vi "ParametrosTeste.View.vi"() -> ()   [LabVIEW 2019]
uses:
  Telas.ctl
  <vilib>/Utility/miscctls.llb/LVStringsAndValuesArrayTypeDef_U16.ctl
  <vilib>/Utility/miscctls.llb/LVPositionTypeDef.ctl
  <vilib>/Utility/miscctls.llb/LVPointTypeDef.ctl
  TelaParametrosTeste/VariaveisParametros.vi
  TelaConfig/Configuracao.Variaveis.vi
  <vilib>/Utility/file.llb/Read Delimited Spreadsheet (DBL).vi
panel:
  out "OndaSelecionada":T1(ring)
  out "TipoGeraçãoSelect":u16(ring) items=["Modo Continuo", "Limitado por tempo", "Ponto por ponto"]
  out "HardwareConfiguration":T3(array[cluster])
  out "ProximaTela":T4
  in  "Tab":enum32{"Page 1", "Page 2"}(tab)
  in  "TabTela":enum32{"PlacaNI", "Geracao1", "Geracao2"}(tab)
  out "Info 2":string
  in  "EntradasAnalogicas":u16(ring) caption="Entrada Analógica:" items=["None"]
  in  "Placas":u16(ring) caption="Placa de aquisição:" items=["None"]
  in  "AddMedicao":bool caption="Adicionar:"
  in  "ListaMedicaoPorta":string[][](table)
  in  "TiposMedicoes":T5(ring) caption="Tipos de Medição:"
  out "GeracaoSelecionada":string
  in  "SelecionarGeracao":bool
  out "UnidadeTempoTeste":string
  in  "TempoTeste":dbl caption="Tempo do teste:"
  in  "TesteOnda":bool
  out "Graph":cluster{"X":dbl, "Y":dbl}[](graph)
  in  "TabOndas":T6(tab)
  in  "InfoContinuo":T7 {"TempRampas" format="%#_g s"}
  in  "InfoInSenoide":T8
  in  "Limpar pontos":bool
  in  "Pasta cvs":path caption="Pasta arquivo cvs:"
  in  "TaxaGeracao":dbl caption="Tempo entre pontos:"
  out "Pontos":dbl[](array[numeric]) caption="Pontos:"
  in  "SelectTipoOnda":T1(ring) caption="Forma de onda:"
  in  "Voltar":bool
  out "Info":string
  in  "BotaoProximaTela":bool
  in  "VoltarTela":bool
  in  "SelecaoGeracao":u16(ring) caption="Seleção forma de geração" items=["Modo Continuo", "Limitado por tempo", "Ponto por ponto"]
  in  "Salvar":bool
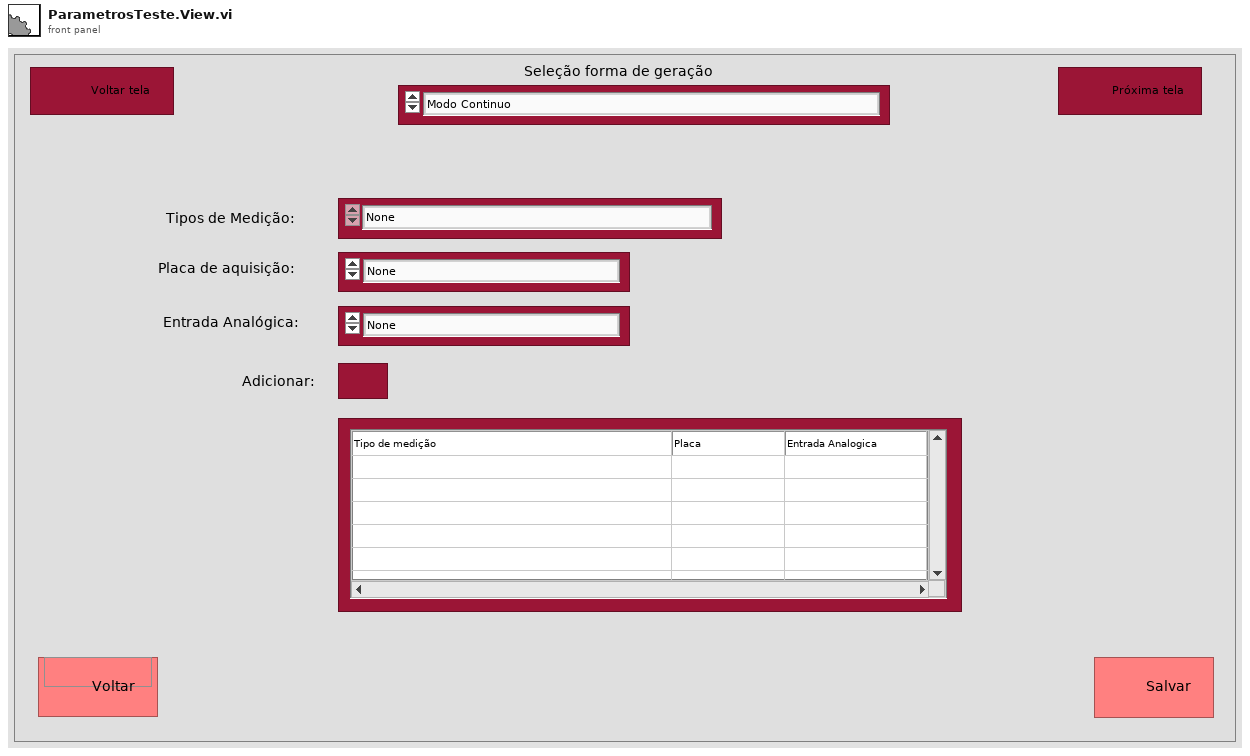
[diagram p1: front panel]
types:
  T1 = enum16{"None", "Continua", "Senoidal", "Quadrada"}
  T2 = typedef "LVStringsAndValuesArrayTypeDef_U16.ctl" = cluster{"String":string, "Value":u16}[]
  T3 = cluster{"ProductCategory":i32, "ProductType":string, "DevIsSimulated":bool, "DigitalInputs":tag[], "DigitalOutputs":tag[], "AnalogInputs":tag[], "AnalogOutputs":tag[], "AnalogInRing":T2}[]
  T4 = typedef "Telas.ctl" = enum16{"Selecao", "Config", "Medicao", "ParametrosTeste"}
  T5 = enum16{"None", "Tensão AeroGerador", "Corrente AeroGerador", "Anemômetro 1", "Anemômetro 2", "Vibração"}
  T6 = enum32{"Contino", "Senoide", "Pontos", "Quadrada"}
  T7 = cluster{"TempRampas":dbl, "PicoMax":dbl, "TextUnidMed":string}
  T8 = cluster{"TexPontosSenoide":string, "RotacaoMinuto":dbl, "PicoMin":dbl, "PicoMax":dbl, "TaxaGeracao":dbl}
  T9 = typedef "LVPositionTypeDef.ctl" = cluster{"Left":i32, "Top":i32}
  T10 = typedef "LVPointTypeDef.ctl" = cluster{"Horizontal":i16, "Vertical":i16}
  T11 = enum16{"None", "Continua", "Senoidal", "Quadrada", "Pontos"}
  T12 = cluster{"ProductCategory":i32, "ProductType":string, "DevIsSimulated":bool, "DigitalInputs":tag[], "DigitalOutputs":tag[], "AnalogInputs":tag[], "AnalogOutputs":tag[], "AnalogInRing":T2}
  T13 = cluster{"Texpontos senoide":string, "AceleracaoMaxima":dbl, "RotacaoMaxMotor":dbl, "PotenciaMotor":dbl, "AceleracaoMaxima 2":dbl}
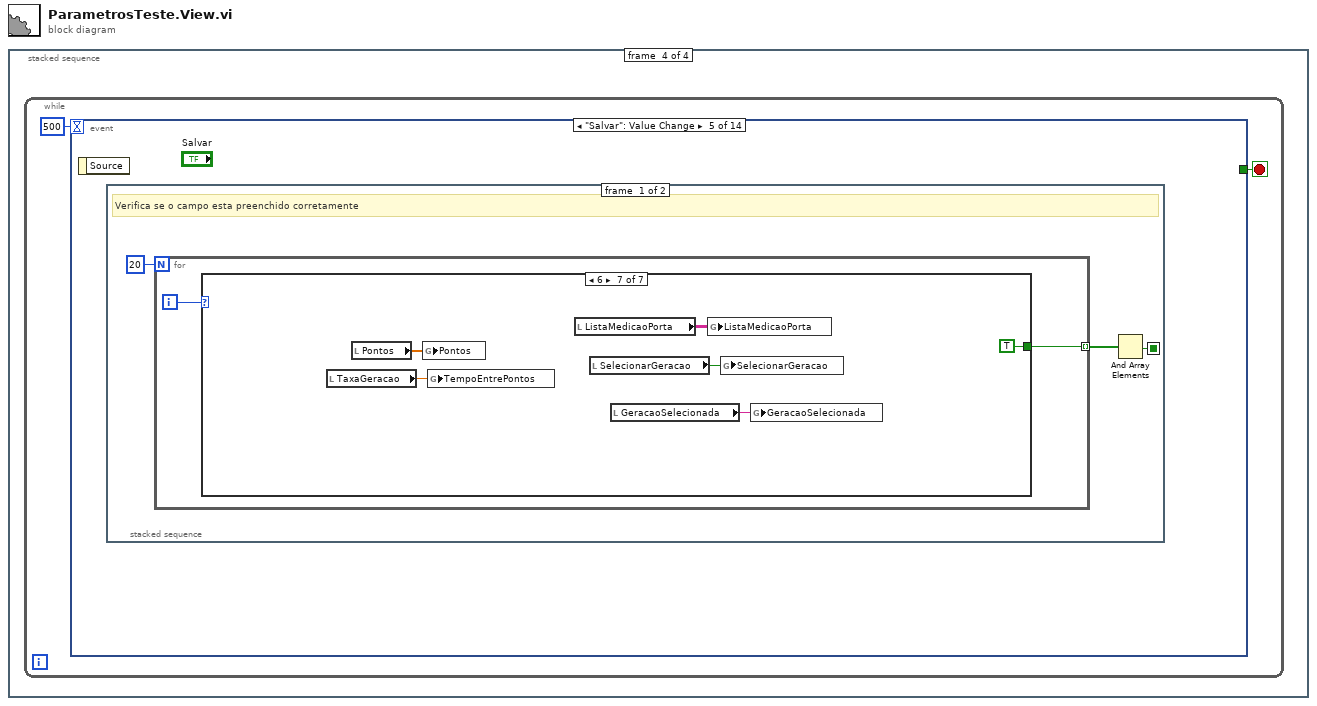
[diagram p0: block diagram]
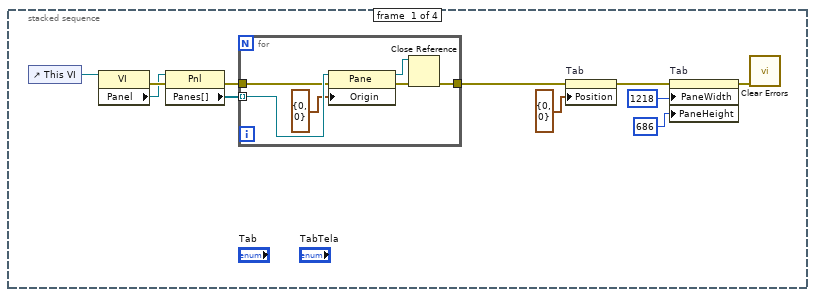
[diagram p2: hidden frame]
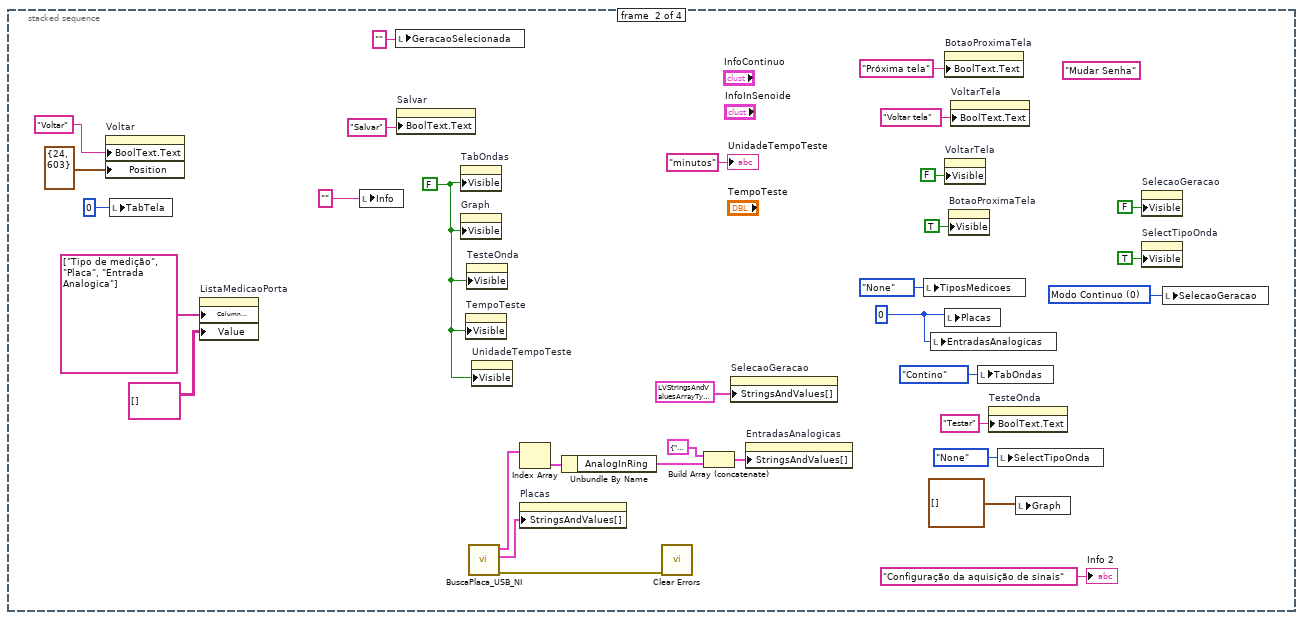
[diagram p3: hidden frame]
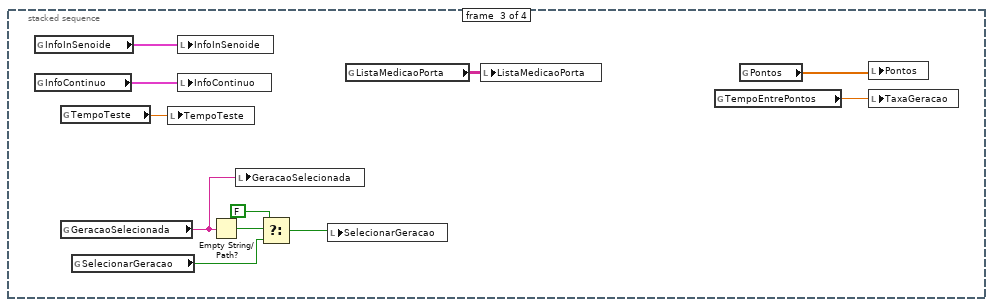
[diagram p4: hidden frame]
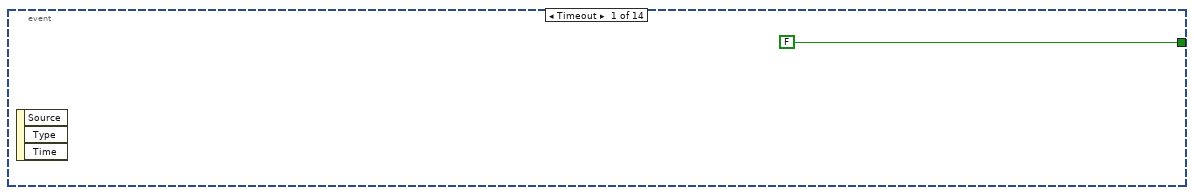
[diagram p5: hidden frame]
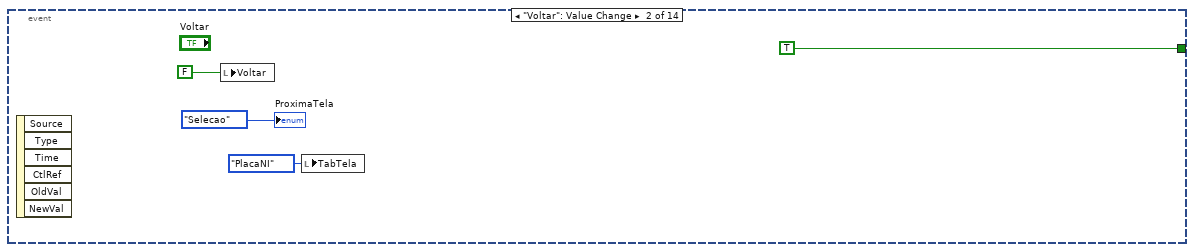
[diagram p6: hidden frame]
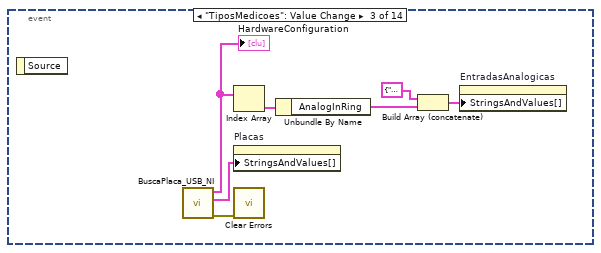
[diagram p7: hidden frame]
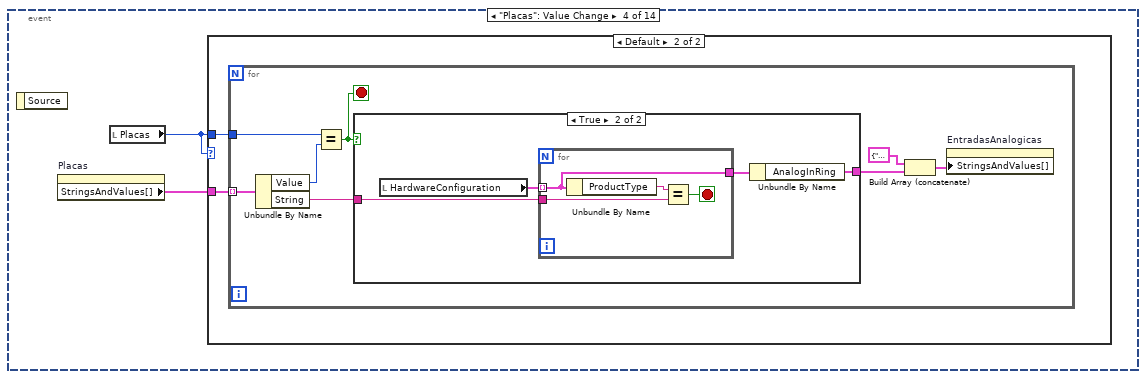
[diagram p8: hidden frame]
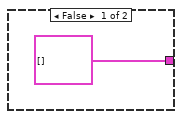
[diagram p10: hidden frame]
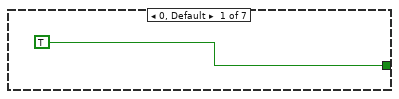
[diagram p11: hidden frame]
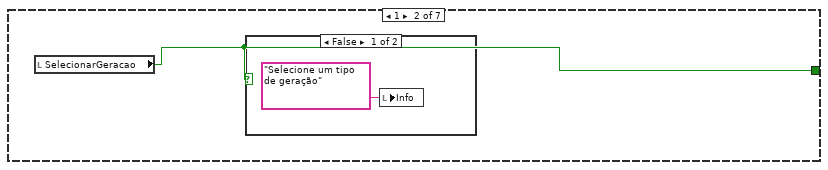
[diagram p12: hidden frame]
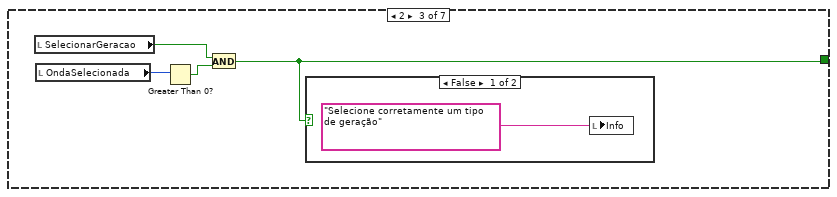
[diagram p14: hidden frame]
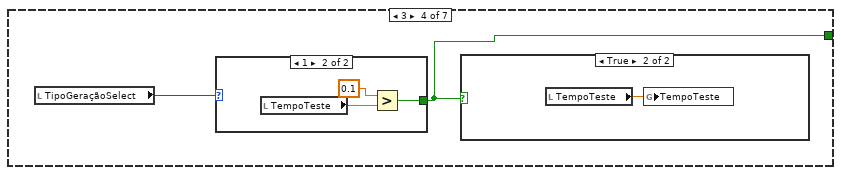
[diagram p16: hidden frame]
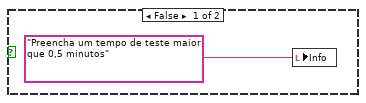
[diagram p17: hidden frame]
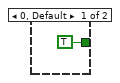
[diagram p18: hidden frame]
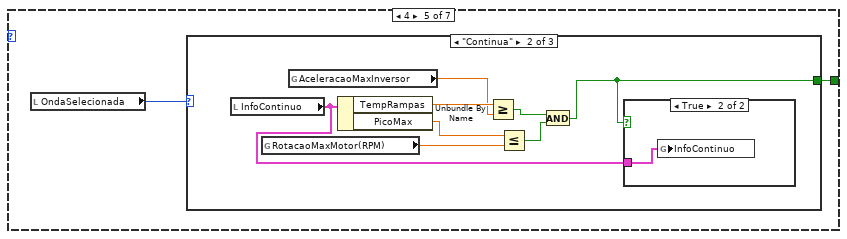
[diagram p19: hidden frame]
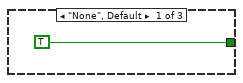
[diagram p20: hidden frame]
diagram:
  n1 = stacked-sequence {
    frame #0 {
      n2 = control-ref of="This VI"() -> (w8:refnum<vi>)
      n3 = property class="VI"(reference=w8) -> (error out=w11:errorcluster, "Panel"=w10:refnum<vi>)  [unwired: 1 in, 1 out]
      n4 = property class="Pnl"(reference=w10, error in=w11) -> (error out=w7:errorcluster, "Panes[]"=w9:refnum<vi>[])  [unwired: 1 out]
      n5 = for {
        tunnel: w9 -> [w17] mode=indexing
        tunnel: w7 -> [w13]
        tunnel: [w12] -> w6
        n6 = property class="Pane"(reference=w17, error in=w13, "Origin"=T10 {"Horizontal"=0, "Vertical"=0}) -> (reference out=w14:refnum<vi>, error out=w15:errorcluster)
        n7 = Close Reference(reference=w14, error in (no error)=w15) -> (error out=w12:errorcluster)
      }
      n8 = property on="Tab" class="TabCtl (strict)"(error in=w6, "Position"=T9 {"Left"=0, "Top"=0}) -> (error out=w5:errorcluster)  [unwired: 1 in, 1 out]
      n9 = property on="Tab" class="TabCtl (strict)"(error in=w5, "PaneWidth"=u32 1218 ("Tab Control Pane Dimension:Width"), "PaneHeight"=u32 686 ("Tab Control Pane Dimension:Height")) -> (error out=w4:errorcluster)  [unwired: 1 in, 1 out]
      n10 = call <vilib>:"Clear Errors.vi"("error in (no error)"=w4) -> ()  [unwired: 5 in, 2 out]
    }
    frame #1 {
      w18 = u16 0 items=["Modo Continuo", "Limitado por tempo", "Ponto por ponto"] ("SelecaoGeracao")
      w25 = FALSE
      w32 = 0
      (unwired) "Mudar Senha" ("Boolean Text.Text")
      n11 = property on="Voltar" class="Bool (strict)"("BoolText.Text"="Voltar" ("Boolean Text.Text"), "Position"=T9 {"Left"=24, "Top"=603}) -> ()  [unwired: 2 in, 2 out]
      n12 = local write "TabTela"(0) -> ()
      n13 = property on="ListaMedicaoPorta" class="Tbl (strict)"("Column Headers[]"=string[] ["Tipo de medição", "Placa", "Entrada Analogica"] ("Column Header Strings[]"), "Value"=string[][] [] ("Item Names")) -> ()  [unwired: 2 in, 2 out]
      n14 = local write "Info"("" ("InfoConfig")) -> ()
      n15 = local write "GeracaoSelecionada"("" ("GeracaoSelecionada")) -> ()
      n16 = property on="Salvar" class="Bool"("BoolText.Text"="Salvar" ("Boolean Text.Text")) -> ()  [unwired: 2 in, 2 out]
      n17 = property on="TabOndas" class="TabCtl (strict)"("Visible"=w25) -> ()  [unwired: 2 in, 2 out]
      n18 = property on="Graph" class="XYGraph (strict)"("Visible"=w25) -> ()  [unwired: 2 in, 2 out]
      n19 = property on="TempoTeste" class="DigNum (strict)"("Visible"=w25) -> ()  [unwired: 2 in, 2 out]
      n20 = property on="TesteOnda" class="Bool"("Visible"=w25) -> ()  [unwired: 2 in, 2 out]
      n21 = call "BuscaPlaca_USB_NI.vi"() -> ("error out"=w40:errorcluster, "PlacasRing"=w37:cluster{"String":string, "Value":u16}[], "HardwareConfiguration"=w42:T3)  [unwired: 9 in]
      n22 = property on="UnidadeTempoTeste" class="Str"("Visible"=w25) -> ()  [unwired: 2 in, 2 out]
      n23 = Index Array(array=w42) -> (element=w41:T12)  [unwired: 1 in]
      n24 = property on="Placas" class="Ring (strict)"("StringsAndValues[]"=w37) -> ()  [unwired: 2 in, 2 out]
      n25 = Unbundle By Name(w41) -> ("AnalogInRing"=w39:T2)
      n26 = call <vilib>:"Clear Errors.vi"("error in (no error)"=w40) -> ()  [unwired: 5 in, 2 out]
      n27 = Build Array (concatenate)(cluster{"String":string, "Value":u16} {"String"="None", "Value"=0}, w39) -> (w38:T2)
      n28 = property on="SelecaoGeracao" class="Ring (strict)"("StringsAndValues[]"=T2 [{"String"="Modo Continuo", "Value"=0}, {"String"="Limitado por tempo", "Value"=1}, {"String"="Ponto por ponto", "Value"=2}] ("Strings And Values []")) -> ()  [unwired: 2 in, 2 out]
      n29 = property on="EntradasAnalogicas" class="Ring (strict)"("StringsAndValues[]"=w38) -> ()  [unwired: 2 in, 2 out]
      n30 = local write "TiposMedicoes"(T5."None" ("TiposMedicoes")) -> ()
      n31 = local write "EntradasAnalogicas"(w32) -> ()
      n32 = property on="BotaoProximaTela" class="Bool"("BoolText.Text"="Próxima tela" ("Boolean Text.Text")) -> ()  [unwired: 2 in, 2 out]
      n33 = property on="VoltarTela" class="Bool"("Visible"=FALSE) -> ()  [unwired: 2 in, 2 out]
      n34 = local write "Placas"(w32) -> ()
      n35 = property on="BotaoProximaTela" class="Bool"("Visible"=TRUE) -> ()  [unwired: 2 in, 2 out]
      n36 = property on="VoltarTela" class="Bool"("BoolText.Text"="Voltar tela" ("Boolean Text.Text")) -> ()  [unwired: 2 in, 2 out]
      n37 = local write "TabOndas"(T6."Contino" ("TabOndas")) -> ()
      n38 = property on="TesteOnda" class="Bool"("BoolText.Text"="Testar" ("Boolean Text.Text")) -> ()  [unwired: 2 in, 2 out]
      n39 = local write "SelectTipoOnda"(T11."None" ("SelectTipoOnda")) -> ()
      n40 = local write "Graph"(cluster{"X":dbl, "Y":dbl}[] [] ("XY Graph")) -> ()
      n41 = property on="SelecaoGeracao" class="Ring (strict)"("Visible"=FALSE) -> ()  [unwired: 2 in, 2 out]
      n42 = property on="SelectTipoOnda" class="Enum (strict)"("Visible"=TRUE) -> ()  [unwired: 2 in, 2 out]
      n43 = local write "SelecaoGeracao"(w18) -> ()
      "UnidadeTempoTeste" <- "minutos" ("UnidadeTempoTeste")
      "Info 2" <- "Configuração da aquisição de sinais" ("Info 2")
    }
    frame #2 {
      n44 = global read "VariaveisParametros.vi" "InfoInSenoide"() -> (w58:T13)
      n45 = global read "VariaveisParametros.vi" "InfoContinuo"() -> (w60:T7)
      n46 = global read "VariaveisParametros.vi" "TempoTeste"() -> (w59:dbl)
      n47 = global read "VariaveisParametros.vi" "GeracaoSelecionada"() -> (w53:string)
      n48 = global read "VariaveisParametros.vi" "SelecionarGeracao"() -> (w56:bool)
      n49 = local write "TempoTeste"(w59) -> ()
      n50 = local write "InfoInSenoide"(w58) -> ()
      n51 = local write "InfoContinuo"(w60) -> ()
      n52 = Empty String/Path?(string/path=w53) -> (empty?=w57:bool)
      n53 = local write "GeracaoSelecionada"(w53) -> ()
      n54 = Select(t=FALSE, s=w57, f=w56) -> (s? t:f=w54:bool)
      n55 = local write "SelecionarGeracao"(w54) -> ()
      n56 = global read "VariaveisParametros.vi" "ListaMedicaoPorta"() -> (w52:string[][])
      n57 = local write "ListaMedicaoPorta"(w52) -> ()
      n58 = global read "VariaveisParametros.vi" "TempoEntrePontos"() -> (w50:dbl)
      n59 = global read "VariaveisParametros.vi" "Pontos"() -> (w51:dbl[])
      n60 = local write "Pontos"(w51) -> ()
      n61 = local write "TaxaGeracao"(w50) -> ()
    }
    frame #3 {
      n62 = while {
        stop <- w61 stop-if-true
        n63 = event shown="[4] \"Salvar\": Value Change" {
          selector: _ -> [_ _ _ _ _ _ _ _ _ _ _ _ _ _]
          dyn-events: _ -> [_ _ _ _ _ _ _ _ _ _ _ _ _ _]
          timeout: 500 -> [_ _ _ _ _ _ _ _ _ _ _ _ _ _]
          tunnel: [FALSE TRUE _ _ _ _ _ _ _ _ _ _ _ _] -> w61
          event Timeout {
            n64 = event-data() -> ()  [unwired: 1 in, 3 out]
          }
          event "Voltar": Value Change {
            n65 = event-data() -> ()  [unwired: 1 in, 6 out]
            n66 = local write "Voltar"(FALSE ("VoltarButton")) -> ()
            n67 = local write "TabTela"(enum32{"PlacaNI", "Geracao1", "Geracao2"}."PlacaNI" ("TabTela")) -> ()
            "ProximaTela" <- Telas."Selecao" ("NextScreen")
          }
          event "TiposMedicoes": Value Change {
            n68 = event-data() -> ()  [unwired: 1 in, 1 out]
            n69 = call "BuscaPlaca_USB_NI.vi"() -> ("error out"=w73:errorcluster, "PlacasRing"=w70:cluster{"String":string, "Value":u16}[], "HardwareConfiguration"=w68:T3)  [unwired: 9 in]
            "HardwareConfiguration" <- w68
            n70 = Index Array(array=w68) -> (element=w74:T12)  [unwired: 1 in]
            n71 = property on="Placas" class="Ring (strict)"("StringsAndValues[]"=w70) -> ()  [unwired: 2 in, 2 out]
            n72 = call <vilib>:"Clear Errors.vi"("error in (no error)"=w73) -> ()  [unwired: 5 in, 2 out]
            n73 = Unbundle By Name(w74) -> ("AnalogInRing"=w72:T2)
            n74 = Build Array (concatenate)(cluster{"String":string, "Value":u16} {"String"="None", "Value"=0}, w72) -> (w71:T2)
            n75 = property on="EntradasAnalogicas" class="Ring (strict)"("StringsAndValues[]"=w71) -> ()  [unwired: 2 in, 2 out]
          }
          event "Placas": Value Change {
            n76 = event-data() -> ()  [unwired: 1 in, 1 out]
            n77 = property on="Placas" class="Ring (strict)"() -> ("StringsAndValues[]"=w76:T2)  [unwired: 2 in, 2 out]
            n78 = local read "Placas"() -> (w75:u16)
            n79 = case shown="Default" w75 {
              tunnel: w76 -> [_ w78]
              tunnel: w75 -> [_ w77]
              frame 0 {
              }
              frame Default {
                n80 = for {
                  tunnel: w78 -> [w86] mode=indexing
                  tunnel: w77 -> [w84]
                  stop <- w83 stop-if-true
                  n81 = Unbundle By Name(w86) -> ("Value"=w85:u16, "String"=w82:string)
                  n82 = Equal?(x=w84, y=w85) -> (x = y?=w83:bool)
                  n83 = case shown="True" w83 {
                    tunnel: w82 -> [_ w90]
                    tunnel: [T2 [] ("AnalogInRing") w88] -> w80
                    frame False {
                    }
                    frame True {
                      n84 = local read "HardwareConfiguration"() -> (w91:T3)
                      n85 = for {
                        tunnel: w91 -> [w93] mode=indexing
                        tunnel: w90 -> [w94]
                        tunnel: [w93] -> w89
                        stop <- w92 stop-if-true
                        n86 = Unbundle By Name(w93) -> ("ProductType"=w95:string)
                        n87 = Equal?(x=w95, y=w94) -> (x = y?=w92:bool)
                      }
                      n88 = Unbundle By Name(w89) -> ("AnalogInRing"=w88:T2)
                    }
                  }
                  n89 = Build Array (concatenate)(cluster{"String":string, "Value":u16} {"String"="None", "Value"=0}, w80) -> (w79:T2)
                  n90 = property on="EntradasAnalogicas" class="Ring (strict)"("StringsAndValues[]"=w79) -> ()  [unwired: 2 in, 2 out]
                }
              }
            }
          }
          event "Salvar": Value Change {
            n91 = event-data() -> ()  [unwired: 1 in, 1 out]
            n92 = stacked-sequence {
              seq-local: [w97 _] -> [_ w140]
              frame #0 {
                # "Verifica se o campo esta preenchido corretamente"
                n93 = for {
                  N: 20 -> [_]
                  tunnel: [w99] -> w98 mode=indexing
                  i -> [w100]
                  n94 = case shown="6" w100 {
                    tunnel: [TRUE w102 w104 w109 w117 TRUE ("SelecionarGeracao") TRUE ("SelecionarGeracao")] -> w99
                    frame 0, Default {
                    }
                    frame 1 {
                      n95 = local read "SelecionarGeracao"() -> (w102:bool)
                      n96 = case shown="False" w102 {
                        frame False {
                          n97 = local write "Info"("Selecione um tipo de geração" ("Info")) -> ()
                        }
                        frame True {
                        }
                      }
                    }
                    frame 2 {
                      n98 = local read "SelecionarGeracao"() -> (w105:bool)
                      n99 = local read "OndaSelecionada"() -> (w107:T1)
                      n100 = Greater Than 0?(x=w107) -> (x > 0?=w106:bool)
                      n101 = And(x=w105, y=w106) -> (x .and. y?=w104:bool)
                      n102 = case shown="False" w104 {
                        frame False {
                          n103 = local write "Info"("Selecione corretamente um tipo de geração" ("Info")) -> ()
                        }
                        frame True {
                        }
                      }
                    }
                    frame 3 {
                      n104 = local read "TipoGeraçãoSelect"() -> (w110:u16)
                      n105 = case shown="1" w110 {
                        tunnel: [TRUE w114] -> w109
                        frame 0, Default {
                        }
                        frame 1 {
                          n106 = local read "TempoTeste"() -> (w116:dbl)
                          n107 = Greater?(x=0.1, y=w116) -> (0:w114:bool)
                        }
                      }
                      n108 = case shown="True" w109 {
                        frame False {
                          n109 = local write "Info"("Preencha um tempo de teste maior que 0,5 minutos" ("Info")) -> ()
                        }
                        frame True {
                          n110 = local read "TempoTeste"() -> (w112:dbl)
                          n111 = global write "VariaveisParametros.vi" "TempoTeste"(w112) -> ()
                        }
                      }
                    }
                    frame 4 {
                      n112 = local read "OndaSelecionada"() -> (w118:T1)
                      n113 = case shown="\"Continua\"" w118 {
                        tunnel: [TRUE w121 TRUE] -> w117
                        frame "None", Default {
                        }
                        frame "Continua" {
                          n114 = local read "InfoContinuo"() -> (w120:T7)
                          n115 = global read "Configuracao.Variaveis.vi" "RotacaoMaxMotor(RPM)"() -> (w124:dbl)
                          n116 = global read "Configuracao.Variaveis.vi" "AceleracaoMaxInversor"() -> (w126:dbl)
                          n117 = Unbundle By Name(w120) -> ("TempRampas"=w127:dbl, "PicoMax"=w125:dbl)
                          n118 = Greater Or Equal?(x=w127, y=w126) -> (x >= y?=w123:bool)
                          n119 = Less Or Equal?(x=w125, y=w124) -> (x <= y?=w122:bool)
                          n120 = And(x=w123, y=w122) -> (x .and. y?=w121:bool)
                          n121 = case shown="True" w121 {
                            tunnel: w120 -> [_ w128]
                            frame False {
                            }
                            frame True {
                              n122 = global write "VariaveisParametros.vi" "InfoContinuo"(w128) -> ()
                            }
                          }
                        }
                        frame "Senoidal" {
                          n123 = local read "InfoInSenoide"() -> (w130:T8)
                          n124 = global write "VariaveisParametros.vi" "InfoInSenoide"(w130) -> ()
                        }
                      }
                    }
                    frame 5 {
                      # "fAZER AS VALIDA钦ES \nE\nADICIONAR NAS VI QUE SALVA\nAS VARIAVEIS"
                      n125 = local read "TipoGeraçãoSelect"() -> (w132:u16)
                      n126 = local read "OndaSelecionada"() -> (w133:T1)
                      n127 = global write "VariaveisParametros.vi" "TipoGeraçãoSelect"(w132) -> ()
                      n128 = global write "VariaveisParametros.vi" "OndaSelecionada"(w133) -> ()
                    }
                    frame 6 {
                      n129 = local read "TaxaGeracao"() -> (w134:dbl)
                      n130 = local read "Pontos"() -> (w135:dbl[])
                      n131 = global write "VariaveisParametros.vi" "Pontos"(w135) -> ()
                      n132 = global write "VariaveisParametros.vi" "TempoEntrePontos"(w134) -> ()
                      n133 = local read "ListaMedicaoPorta"() -> (w136:string[][])
                      n134 = local read "SelecionarGeracao"() -> (w138:bool)
                      n135 = local read "GeracaoSelecionada"() -> (w139:string)
                      n136 = global write "VariaveisParametros.vi" "ListaMedicaoPorta"(w136) -> ()
                      n137 = global write "VariaveisParametros.vi" "SelecionarGeracao"(w138) -> ()
                      n138 = global write "VariaveisParametros.vi" "GeracaoSelecionada"(w139) -> ()
                    }
                  }
                }
                n139 = And Array Elements(Boolean array=w98) -> (logical AND=w97:bool)
              }
              frame #1 {
                n140 = case shown="True" w140 {
                  frame False {
                    # "Algo não esta preenchido corretamente"
                    "Info" <- "Erro: Falta preencher algum campo corretamente" ("InfoConfig")
                  }
                  frame True {
                    # "Preenchimento correto dos campos"
                    n141 = call "Configuracao.Escrita.vi"() -> ("error out"=w142:errorcluster)  [unwired: 11 in]
                    n142 = case shown="No Error" w142 {
                      tunnel: ["Informações salvas" ("InfoConfig") "Erro ao salvar as variavies" ("InfoConfig")] -> w143
                      frame No Error {
                      }
                      frame Error {
                      }
                    }
                    n143 = local write "Info"(w143) -> ()
                  }
                }
              }
            }
          }
          event "AddMedicao": Value Change {
            (unwired) T5."None" ("TiposMedicoes")
            n144 = event-data() -> ()  [unwired: 1 in, 1 out]
            n145 = Greater Than 0?(x="TiposMedicoes") -> (x > 0?=w146:bool)
            n146 = Greater Than 0?(x="Placas") -> (x > 0?=w149:bool)
            n147 = Greater Than 0?(x="EntradasAnalogicas") -> (x > 0?=w150:bool)
            n148 = Compound Arithmetic op=AND(w146, w149, w150) -> (w148:bool)
            n149 = case shown="True" w148 {
              frame False {
                # "Memoria vazia. Erro"
              }
              frame True {
                # "Registra a limpa variaveis"
                n150 = property on="EntradasAnalogicas" class="Ring (strict)"() -> ("RingText.Text"=w154:string)  [unwired: 2 in, 2 out]
                n151 = property on="TiposMedicoes" class="Enum (strict)"() -> ("RingText.Text"=w156:string)  [unwired: 2 in, 2 out]
                n152 = property on="Placas" class="Ring (strict)"() -> ("RingText.Text"=w155:string)  [unwired: 2 in, 2 out]
                n153 = Build Array(w156, w155, w154) -> (w153:string[])
                n154 = Insert Into Array(array="ListaMedicaoPorta", new element=w153) -> (w158:string[][])  [unwired: 2 in]
                n155 = local write "ListaMedicaoPorta"(w158) -> ()
              }
            }
          }
          event "BotaoProximaTela": Value Change {
            n156 = event-data() -> ()  [unwired: 1 in, 1 out]
            n157 = local read "TabTela"() -> (w163:enum32{"PlacaNI", "Geracao1", "Geracao2"})
            n158 = Increment(x=w163) -> (x+1=w159:enum32{"PlacaNI", "Geracao1", "Geracao2"})
            n159 = case shown="\"PlacaNI\"" w159 {
              tunnel: [TRUE FALSE TRUE] -> w162
              tunnel: [TRUE TRUE FALSE] -> w161
              tunnel: [TRUE FALSE TRUE] -> w160
              frame Default {
              }
              frame "PlacaNI" {
                n160 = property on="SelecaoGeracao" class="Ring (strict)"("Val(Sgnl)"=u16 0 ("Value (Signaling)")) -> ()  [unwired: 2 in, 2 out]
              }
              frame "Geracao2" {
              }
            }
            n161 = local write "TabTela"(w159) -> ()
            n162 = property on="VoltarTela" class="Bool"("Visible"=w162) -> ()  [unwired: 2 in, 2 out]
            n163 = property on="ProximaTela" class="Bool"("Visible"=w161) -> ()  [unwired: 2 in, 2 out]
            n164 = property on="SelecaoGeracao" class="Ring (strict)"("Visible"=w160) -> ()  [unwired: 2 in, 2 out]
          }
          event "VoltarTela": Value Change {
            n165 = event-data() -> ()  [unwired: 1 in, 6 out]
            n166 = local read "TabTela"() -> (w178:enum32{"PlacaNI", "Geracao1", "Geracao2"})
            n167 = Decrement(x=w178) -> (x-1=w174:enum32{"PlacaNI", "Geracao1", "Geracao2"})
            n168 = case shown="Default" w174 {
              tunnel: [TRUE FALSE TRUE] -> w177
              tunnel: [TRUE TRUE FALSE] -> w176
              tunnel: [TRUE FALSE TRUE] -> w175
              frame Default {
              }
              frame "PlacaNI" {
              }
              frame "Geracao2" {
              }
            }
            n169 = local write "TabTela"(w174) -> ()
            n170 = property on="VoltarTela" class="Bool"("Visible"=w177) -> ()  [unwired: 2 in, 2 out]
            n171 = property on="ProximaTela" class="Bool"("Visible"=w176) -> ()  [unwired: 2 in, 2 out]
            n172 = property on="SelecaoGeracao" class="Ring (strict)"("Visible"=w175) -> ()  [unwired: 2 in, 2 out]
          }
          event "SelecaoGeracao": Value Change {
            n173 = event-data() -> ()  [unwired: 1 in, 1 out]
            n174 = property on="SelecaoGeracao" class="Ring (strict)"() -> ("Value"=w189:u16)  [unwired: 2 in, 2 out]
            n175 = case shown="2, Default" w189 {
              tunnel: [enum32{"PlacaNI", "Geracao1", "Geracao2"}."Geracao1" ("TabTela") enum32{"PlacaNI", "Geracao1", "Geracao2"}."Geracao1" ("TabTela") enum32{"PlacaNI", "Geracao1", "Geracao2"}."Geracao1" ("TabTela")] -> w194
              tunnel: [FALSE FALSE TRUE] -> w193
              tunnel: [FALSE TRUE TRUE] -> w191
              tunnel: [w207 FALSE FALSE] -> w188
              frame 2, Default {
                w207 = TRUE
                n176 = local write "TabOndas"(T6."Pontos" ("TabOndas")) -> ()
                n177 = local write "SelectTipoOnda"(T1."None" ("SelectTipoOnda")) -> ()
                n178 = property on="TabOndas" class="TabCtl (strict)"("Visible"=w207) -> ()  [unwired: 2 in, 2 out]
                n179 = property on="Graph" class="XYGraph (strict)"("Visible"=w207) -> ()  [unwired: 2 in, 2 out]
                n180 = property on="TesteOnda" class="Bool"("Visible"=w207) -> ()  [unwired: 2 in, 2 out]
              }
              frame 0 {
              }
              frame 1 {
              }
            }
            n181 = local write "TabTela"(w194) -> ()
            n182 = property on="TempoTeste" class="DigNum (strict)"("Visible"=w193) -> ()  [unwired: 2 in, 2 out]
            n183 = property on="SelectTipoOnda" class="Enum (strict)"("Visible"=w191) -> ()  [unwired: 2 in, 2 out]
            n184 = local read "SelecionarGeracao"() -> (w192:bool)
            n185 = local read "TabOndas"() -> (w190:T6)
            n186 = case shown="False" w192 {
              tunnel: w188 -> [w202 _]
              frame False {
                n187 = property on="SelectTipoOnda" class="Enum (strict)"() -> ("RingText.Text"=w201:string)  [unwired: 2 in, 2 out]
                n188 = property on="SelecaoGeracao" class="Ring (strict)"() -> ("RingText.Text"=w205:string)  [unwired: 2 in, 2 out]
                n189 = Select(t="Pontos", s=w202, f=w201) -> (s? t:f=w199:string)
                n190 = Concatenate Strings(w205, "\r", "Onda: " ("string"), w199) -> (w206:string)
                n191 = local write "GeracaoSelecionada"(w206) -> ()
              }
              frame True {
              }
            }
            n192 = case shown="\"Pontos\"" w190 {
              tunnel: w189 -> [_ w197]
              frame Default {
              }
              frame "Pontos" {
                n193 = Not Equal?(x=w197, y=u16 2) -> (x != y?=w195:bool)
                n194 = case shown="True" w195 {
                  frame False {
                  }
                  frame True {
                    n195 = property on="SelectTipoOnda" class="Enum (strict)"("Val(Sgnl)"=T1."None" ("Value (Signaling)")) -> ()  [unwired: 2 in, 2 out]
                  }
                }
              }
            }
          }
          event "SelectTipoOnda": Value Change {
            n196 = event-data() -> ()  [unwired: 1 in, 1 out]
            n197 = case shown="\"Continua\"" "SelectTipoOnda" {
              tunnel: [FALSE TRUE TRUE TRUE] -> w223
              tunnel: [T6."Contino" ("TabOndas") T6."Contino" ("TabOndas") T6."Senoide" ("TabOndas") T6."Quadrada" ("TabOndas")] -> w221
              frame "None", Default {
              }
              frame "Continua" {
              }
              frame "Senoidal" {
              }
              frame "Quadrada" {
              }
            }
            n198 = property on="TabOndas" class="TabCtl (strict)"("Visible"=w223) -> ()  [unwired: 2 in, 2 out]
            n199 = property on="Graph" class="XYGraph (strict)"("Visible"=w223) -> ()  [unwired: 2 in, 2 out]
            n200 = property on="TesteOnda" class="Bool"("Visible"=w223) -> ()  [unwired: 2 in, 2 out]
            n201 = local write "TabOndas"(w221) -> ()
            n202 = local read "SelecionarGeracao"() -> (w222:bool)
            n203 = case shown="False" w222 {
              frame False {
                n204 = property on="SelectTipoOnda" class="Enum (strict)"() -> ("RingText.Text"=w228:string)  [unwired: 2 in, 2 out]
                n205 = property on="SelecaoGeracao" class="Ring (strict)"() -> ("RingText.Text"=w226:string)  [unwired: 2 in, 2 out]
                n206 = Concatenate Strings(w226, "\r", "Onda: " ("string"), w228) -> (→"GeracaoSelecionada":string)
              }
              frame True {
              }
            }
          }
          event "TesteOnda": Value Change {
            n207 = event-data() -> ()  [unwired: 1 in, 6 out]
            n208 = case shown="\"Senoide\"" "TabOndas" {
              tunnel: [cluster{"X":dbl, "Y":dbl}[] [] ("XY Graph") w241 w245] -> w238
              frame Default {
              }
              frame "Contino" {
                n209 = local read "InfoContinuo"() -> (w244:T7)
                n210 = Unbundle By Name(w244) -> ("PicoMax"=w243:dbl, "TempRampas"=w242:dbl)
                n211 = call "CalculoTesteOndaContinua_Validacao.vi"("TempoRampa"=w242, "PicoMax"=w243) -> ("XY Graph"=w241:cluster{"X":dbl, "Y":dbl}[])  [unwired: 9 in]
              }
              frame "Senoide" {
                n212 = local read "InfoInSenoide"() -> (w250:T8)
                n213 = Unbundle By Name(w250) -> ("PicoMax"=w249:dbl, "PicoMin"=w248:dbl, "RotacaoMinuto"=w247:dbl, "TaxaGeracao"=w246:dbl)
                n214 = call "CalculoTesteSenoide_Validacao.vi"("Taxa de geração"=w246, "Rotações por minuto"=w247, "Min"=w248, "Max"=w249) -> ("XY Graph"=w245:cluster{"X":dbl, "Y":dbl}[])  [unwired: 7 in]
              }
            }
            "Graph" <- w238
          }
          event "SelecionarGeracao": Value Change {
            n215 = event-data() -> ()  [unwired: 1 in, 6 out]
            n216 = local read "SelecaoGeracao"() -> (w258:u16)
            n217 = Equal?(x=w258, y=u16 2) -> (x = y?=w256:bool)
            n218 = case shown="True" "SelecionarGeracao" {
              tunnel: [u32 0 ("NumItems") w267] -> w251
              tunnel: [u32 0 ("NumItems") w266] -> w252
              frame False {
              }
              frame True {
                n219 = property on="SelectTipoOnda" class="Enum (strict)"() -> ("Value"=w266:T1)  [unwired: 2 in, 2 out]
                n220 = property on="SelecaoGeracao" class="Ring (strict)"() -> ("Value"=w267:u16)  [unwired: 2 in, 2 out]
              }
            }
            "TipoGeraçãoSelect" <- w251
            "OndaSelecionada" <- w252
            n221 = property on="SelectTipoOnda" class="Enum (strict)"() -> ("RingText.Text"=w255:string)  [unwired: 2 in, 2 out]
            n222 = Select(t="Pontos", s=w256, f=w255) -> (s? t:f=w253:string)
            n223 = property on="SelecaoGeracao" class="Ring (strict)"() -> ("RingText.Text"=w262:string)  [unwired: 2 in, 2 out]
            n224 = Concatenate Strings(w262, "\r", "Onda: " ("string"), w253) -> (w261:string)
            n225 = local write "GeracaoSelecionada"(w261) -> ()
          }
          event "Pasta cvs": Value Change {
            n226 = event-data() -> ()  [unwired: 1 in, 6 out]
            n227 = call-poly <vilib>:"Read Delimited Spreadsheet.vi"("file path (dialog if empty)"="Pasta cvs") -> ("all rows"=w269:dbl[][])  [unwired: 9 in, 5 out]
            n228 = Index Array(array=w269, index (col)=0 ("disabled index (col)")) -> (element=→"Pontos":dbl[])  [unwired: 1 in]
          }
          event "Limpar pontos": Value Change {
            n229 = event-data() -> ()  [unwired: 1 in, 6 out]
            n230 = local write "Pontos"(dbl[] [] ("Pontos")) -> ()
            n231 = local write "Pasta cvs"(path "" ("Pasta cvs")) -> ()
            n232 = local write "TaxaGeracao"(0.0 ("TaxaGeracao")) -> ()
          }
        }
      }
    }
  }
